vi "2283_solenoids.vi"(11 "feeder":bool) -> (2 "solenoidCorto":T1=enum."Reverse", 3 "solenoidLargo":T1=enum."Reverse")   [LabVIEW 2015]
uses:
  <vilib>/Rock Robotics/WPI/Solenoid/WPI_SolenoidValue.ctl
  TypeDefs/estadosFeeder.ctl
  Globales/Feeder Disponible Global.vi
  Globales/Catapulta Disponible Global.vi
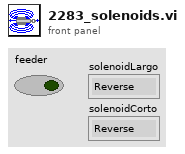
[diagram p1: front panel]
types:
  T1 = typedef "WPI_SolenoidValue.ctl" = enum16{"Off", "On", "Forward", "Reverse"}
  T2 = typedef "estadosFeeder.ctl" = enum16{"regreso3", "regreso2", "regreso1", "afuera2", "afuera1"}
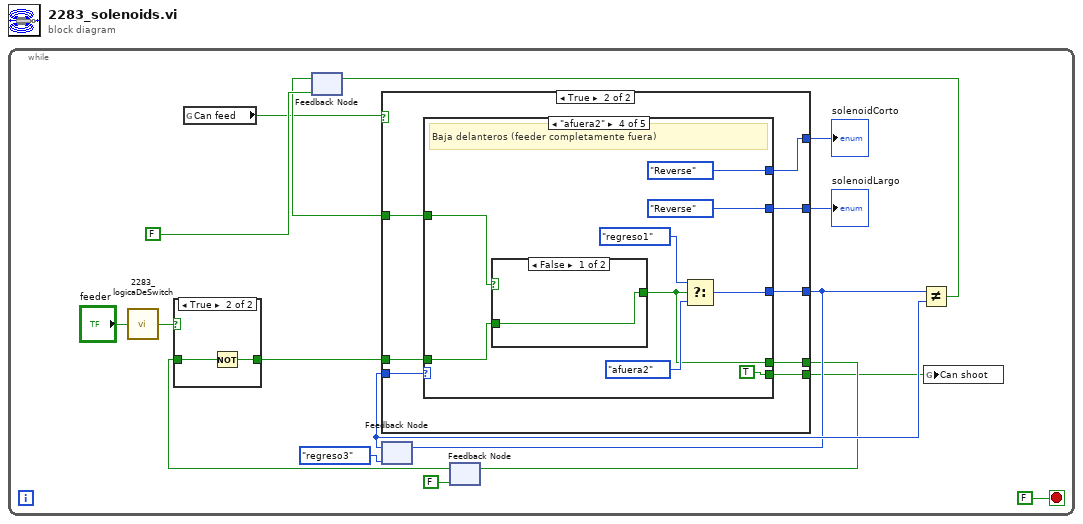
[diagram p0: block diagram]
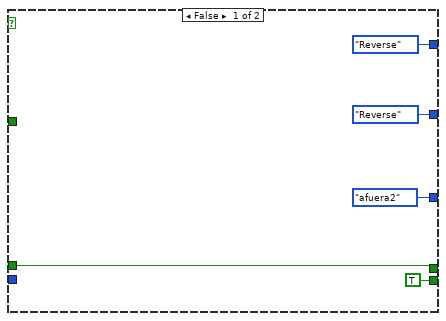
[diagram p2: hidden frame]
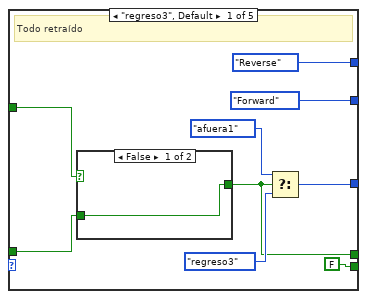
[diagram p3: hidden frame]
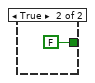
[diagram p4: hidden frame]
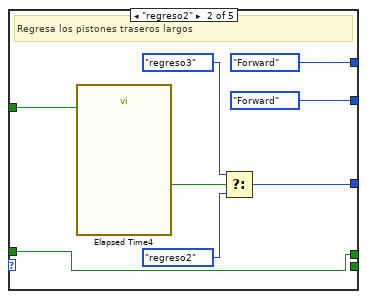
[diagram p5: hidden frame]
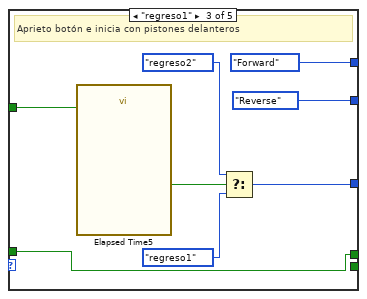
[diagram p6: hidden frame]
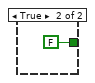
[diagram p7: hidden frame]
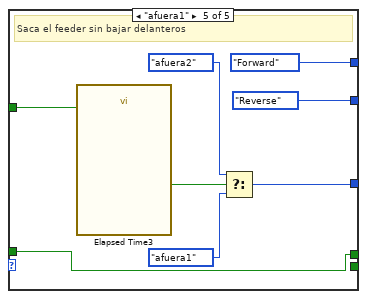
[diagram p8: hidden frame]
diagram:
  n1 = while {
    stop <- FALSE stop-if-true
    n2 = call "2283_logicaDeSwitch.vi"("Input"="feeder") -> ("Output"=w13:bool)
    n3 = global read "Feeder Disponible Global.vi" "Can feed"() -> (w2:bool)
    n4 = feedback #1(FALSE) -> (w6:bool)
    n5 = feedback #2(estadosFeeder."regreso3") -> (w9:T2)
    n6 = feedback #3(FALSE) -> (w12:bool)
    n7 = case shown="True" w13 {
      tunnel: [w77 w79] -> w5
      tunnel: w12 -> [w77 w78]
      frame False {
      }
      frame True {
        n8 = Not(x=w78) -> (.not. x?=w79:bool)
      }
    }
    n9 = case shown="True" w2 {
      tunnel: [WPI_SolenoidValue."Reverse" ("solenoidCorto") w30] -> w16
      tunnel: [WPI_SolenoidValue."Reverse" ("solenoidCorto") w29] -> w15
      tunnel: w9 -> [_ w28]
      tunnel: [estadosFeeder."afuera2" w27] -> w8
      tunnel: w6 -> [_ w26]
      tunnel: w5 -> [w18 w25]
      tunnel: [w18 w24] -> w4
      tunnel: [TRUE w23] -> w3
      frame False {
      }
      frame True {
        n10 = case shown="\"afuera2\"" w28 {
          tunnel: [w39 w45 w54 w62 w72] -> w27
          tunnel: [WPI_SolenoidValue."Reverse" ("solenoidCorto") WPI_SolenoidValue."Forward" ("solenoidCorto") WPI_SolenoidValue."Forward" ("solenoidCorto") WPI_SolenoidValue."Reverse" ("solenoidCorto") WPI_SolenoidValue."Forward" ("solenoidCorto")] -> w30
          tunnel: [WPI_SolenoidValue."Forward" ("solenoidCorto") WPI_SolenoidValue."Forward" ("solenoidCorto") WPI_SolenoidValue."Reverse" ("solenoidCorto") WPI_SolenoidValue."Reverse" ("solenoidCorto") WPI_SolenoidValue."Reverse" ("solenoidCorto")] -> w29
          tunnel: w25 -> [w33 w42 w50 w60 w69]
          tunnel: w26 -> [w34 w43 w51 w61 w70]
          tunnel: [w31 w42 w50 w58 w69] -> w24
          tunnel: [FALSE _ _ TRUE _] -> w23
          frame "regreso3", Default {
            # "Todo retraído"
            n11 = case shown="False" w34 {
              tunnel: [w40 FALSE] -> w31
              tunnel: w33 -> [w40 _]
              frame False {
              }
              frame True {
              }
            }
            n12 = Select(t=estadosFeeder."afuera1", s=w31, f=estadosFeeder."regreso3") -> (s? t:f=w39:T2)
          }
          frame "regreso2" {
            # "Regresa los pistones traseros largos"
            n13 = call "Elapsed Time4"("Reset"=w43) -> ("Time has Elapsed"=w44:bool)  [unwired: 11 in, 7 out]
            n14 = Select(t=estadosFeeder."regreso3", s=w44, f=estadosFeeder."regreso2") -> (s? t:f=w45:T2)
          }
          frame "regreso1" {
            # "Aprieto botón e inicia con pistones delanteros"
            n15 = call "Elapsed Time5"("Reset"=w51) -> ("Time has Elapsed"=w52:bool)  [unwired: 11 in, 7 out]
            n16 = Select(t=estadosFeeder."regreso2", s=w52, f=estadosFeeder."regreso1") -> (s? t:f=w54:T2)
          }
          frame "afuera2" {
            # "Baja delanteros (feeder completamente fuera)"
            n17 = case shown="False" w61 {
              tunnel: [w67 FALSE] -> w58
              tunnel: w60 -> [w67 _]
              frame False {
              }
              frame True {
              }
            }
            n18 = Select(t=estadosFeeder."regreso1", s=w58, f=estadosFeeder."afuera2") -> (s? t:f=w62:T2)
          }
          frame "afuera1" {
            # "Saca el feeder sin bajar delanteros"
            n19 = call "Elapsed Time3"("Reset"=w70) -> ("Time has Elapsed"=w71:bool)  [unwired: 11 in, 7 out]
            n20 = Select(t=estadosFeeder."afuera2", s=w71, f=estadosFeeder."afuera1") -> (s? t:f=w72:T2)
          }
        }
      }
    }
    "solenoidLargo" <- w15
    "solenoidCorto" <- w16
    n21 = feedback-in #2(w8) -> ()
    n22 = feedback-in #3(w4) -> ()
    n23 = Not Equal?(x=w8, y=w9) -> (x != y?=w7:bool)
    n24 = feedback-in #1(w7) -> ()
    n25 = global write "Catapulta Disponible Global.vi" "Can shoot"(w3) -> ()
  }
